vi "PTSequencer.load settings.vi"(0 "i ref in":refnum<vi>, 2 "path":string, 3 "ms timeout (10000)":i32=10000, 5 "error in (no error)":errorcluster) -> (14 "i ref out":refnum<vi>, 17 "timed out":bool, 19 "error out":errorcluster)   [LabVIEW 2014, in "PTSequencer.lvlib"]
uses:
  PTSequencer.lvlib
  <vilib>/Utility/xml.llb/Read From XML File(string).vi
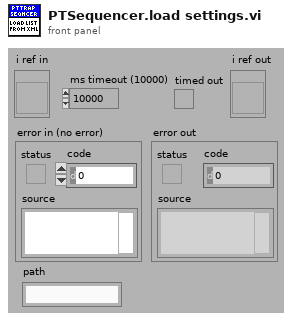
[diagram p1: front panel]
types:
  T1 = typedef "PTSequencer.lvlib/PTSequencer.i attribute.ctl" = cluster{"subsequence":bool, "mode":T2, "i step":i32, "nofLoops":i32, "i loop":i32, "Running":bool, "Paused":bool, "step done":bool, "loop done":bool, "seq done":bool, "DIM IDs":cluster{"step done":i32, "loop done":i32, "seq done":i32, "i step":i32, "i loop":i32}, "use stop conditions":bool, "stop conditions":T3[], "Step List":T5[], "DIM subsriptions":string[], "stop cond indexes":i32[], "step cond indexes":cluster{"step condition IDs":cluster{"step ID":i32, "condition ID":i32}[]}[], "Delay Start Time":timestamp, "status":string, "stopping":bool}
  T2 = typedef "PTSequencer.lvlib/PTSequencer.mode.ctl" = enum16{"single", "loop", "for loop"}
  T3 = typedef "PTSequencer.lvlib/PTSequencer.DIM service condition.ctl" = cluster{"DIM service":string, "descr":string, "nomValue":T4, "actValue":T4, "matched":bool, "DIM Status":cluster{"no link":bool, "quality":i32, "Time Stamp":timestamp}}
  T4 = typedef "CoreDefs.rawDataType.ctl" = i8[]
  T5 = typedef "PTSequencer.lvlib/PTSequencer.step.ctl" = cluster{"description":string, "object parameters":cluster{"object":string, "selector":string, "descriptor":string, "data":T4, "subsequence":bool, "call mode":enum16{"Simple DIM", "Synchronous"}, "data in":T4}, "result action":cluster{"check":bool, "passed":enum16{"Next", "Previous", "Repeat", "Jump"}, "failed":enum16{"Next", "Previous", "Repeat", "Jump"}, "jumpID_passed":i32, "jumpID_failed":i32}, "conditions":T3[], "fulfilled ":bool, "use delay":bool, "delay time (s)":dbl, "ID":i32}
  T6 = cluster{"use stop conditions":bool, "stop conditions":T3[], "Step List":T5[]}
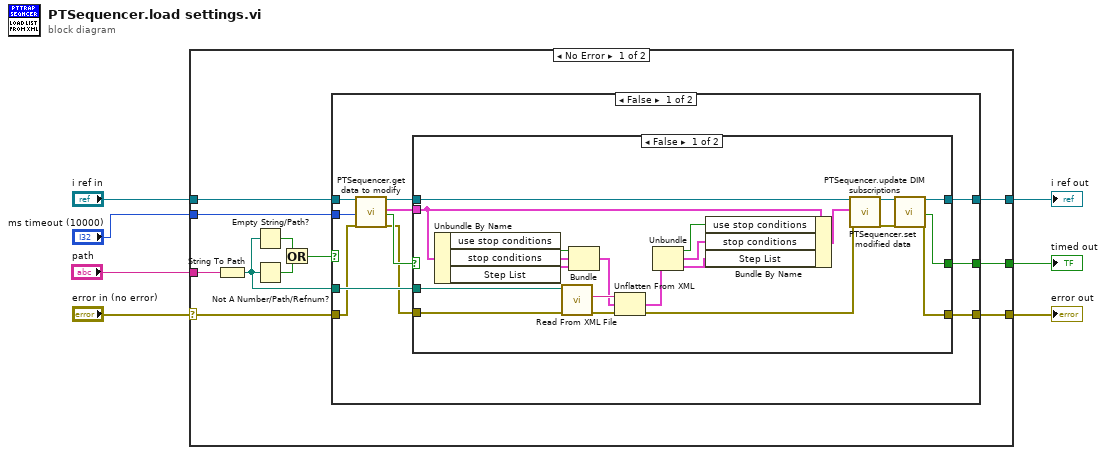
[diagram p0: block diagram]
diagram:
  n1 = case shown="No Error" "error in (no error)" {
    selector: "error in (no error)" -> [w9 w56]
    tunnel: "i ref in" -> [w18 w57]
    tunnel: [w16 w57] -> w5
    tunnel: [w8 w56] -> w4
    tunnel: "ms timeout (10000)" -> [w17 _]
    tunnel: [w15 _] -> w2
    tunnel: "path" -> [w14 _]
    frame No Error {
      n2 = String To Path(string=w14) -> (path=w10:path)
      n3 = Empty String/Path?(string/path=w10) -> (empty?=w13:bool)
      n4 = Not A Number/Path/Refnum?(number/path/refnum=w10) -> (NaN/Path/Refnum?=w12:bool)
      n5 = Or(x=w13, y=w12) -> (x .or. y?=w11:bool)
      n6 = case shown="False" w11 {
        tunnel: w18 -> [w29 w54]
        tunnel: w17 -> [w25 _]
        tunnel: [w24 w54] -> w16
        tunnel: [w23 _] -> w15
        tunnel: w10 -> [w22 _]
        tunnel: w9 -> [w21 w55]
        tunnel: [w19 w55] -> w8
        frame False {
          n7 = call "PTSequencer.get data to modify.vi"("i ref in"=w29, "ms timeout (10000)"=w25, "error in (no error)"=w21) -> ("i ref out"=w28:refnum<vi>, "i attribute"=w27:T1, "timed out"=w26:bool, "error out"=w20:errorcluster)  [unwired: 13 in]
          n8 = case shown="False" w26 {
            selector: w26 -> [_ w52]
            tunnel: w28 -> [w50 w53]
            tunnel: w27 -> [w39 _]
            tunnel: [w31 w53] -> w24
            tunnel: [w30 w52] -> w23
            tunnel: w22 -> [w46 _]
            tunnel: w20 -> [w45 w51]
            tunnel: [w32 w51] -> w19
            frame False {
              n9 = Unbundle By Name(w39) -> ("use stop conditions"=w49:bool, "stop conditions"=w48:T3[], "Step List"=w47:T5[])
              n10 = call-poly <vilib>:"Read From XML File.vi"("error in (no error)"=w45, "XML File Path"=w46) -> ("error out"=w44:errorcluster, "XML Elements"=w42:string)  [unwired: 7 in, 1 out]
              n11 = Bundle("use stop conditions"=w49, "stop conditions"=w48, "Step List"=w47) -> (w41:T6)  [unwired: 1 in]
              n12 = Unflatten From XML(xml string=w42, type=w41, error in (no error)=w44) -> (value=w40:T6, error out=w43:errorcluster)
              n13 = Unbundle(w40) -> ("use stop conditions"=w38:bool, "stop conditions"=w37:T3[], "Step List"=w36:T5[])
              n14 = Bundle By Name(cluster=w39, "use stop conditions"=w38, "stop conditions"=w37, "Step List"=w36) -> (w35:T1)
              n15 = call "PTSequencer.set modified data.vi"("i ref in"=w50, "CLASS.i attribute"=w35, "error in (no error)"=w43) -> ("i ref out"=w34:refnum<vi>, "error out"=w33:errorcluster)  [unwired: 15 in]
              n16 = call "PTSequencer.update DIM subscriptions.vi"("i ref in"=w34, "error in"=w33) -> ("i ref out"=w31:refnum<vi>, "timed out"=w30:bool, "error out"=w32:errorcluster)  [unwired: 15 in]
            }
            frame True {
            }
          }
        }
        frame True {
        }
      }
    }
    frame Error {
    }
  }
  "error out" <- w4
  "i ref out" <- w5
  "timed out" <- w2
